vi "onHttpPut (Buffer).vi"(6 "timeout":i32=10000, 7 "output file":path, 8 "error in":errorcluster, 9 "buffer":string, 10 "url":string, 11 "http-method in":refnum<class "http-client.lvclass">) -> (0 "error out":errorcluster, 1 "body":string, 2 "headers":string, 3 "http-method out":refnum<class "http-client.lvclass">)   [LabVIEW 2020, in "REST Client.lvlib" / "http-client.lvclass"]
uses:
  http-client.lvclass
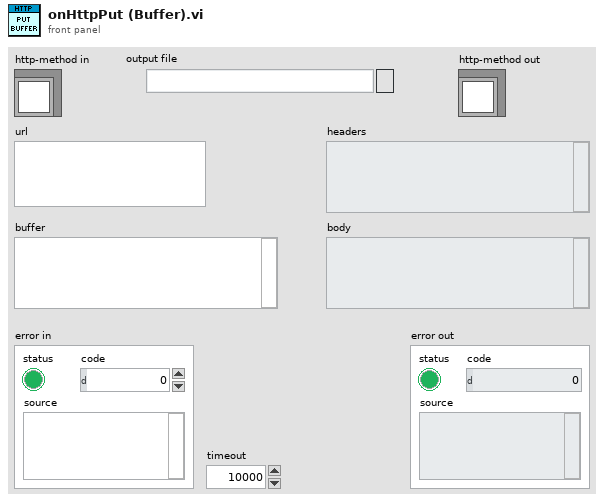
[diagram p1: front panel]
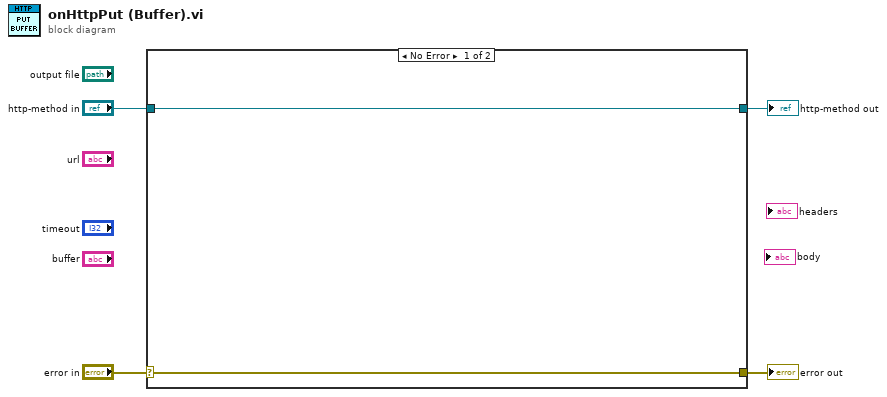
[diagram p0: block diagram]
diagram:
  n1 = case shown="No Error" "error in" {
    selector: "error in" -> [w5 w8]
    tunnel: [w5 w8] -> w3
    tunnel: [w6 w7] -> w1
    tunnel: "http-method in" -> [w6 w7]
    frame No Error {
    }
    frame Error {
    }
  }
  "error out" <- w3
  "http-method out" <- w1
